vi "Read Debug Data.vi"(8 "error in (no error)":errorcluster, 11 "Debugger In":refnum<class "Debugger.lvclass">) -> (0 "error out":errorcluster, 2 "Data Log":refnum<class "Debug Data.lvclass">[](array[class]), 3 "Debugger Out":refnum<class "Debugger.lvclass">)   [LabVIEW 2020, in "Debugger.lvclass"]
uses:
  Debugger.lvclass
  Debug Data/Debug Data.lvclass
  Debug Log/Debug Log.lvclass/Debug Log.ctl
  Debug Log/Read Unfiltered Log Content.vi
  Filter/Filter.lvclass
  Debugger.lvclass/Debugger.ctl
  Debug Log/Debug Log.lvclass
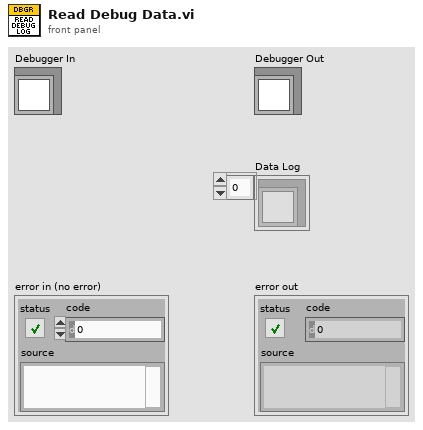
[diagram p1: front panel]
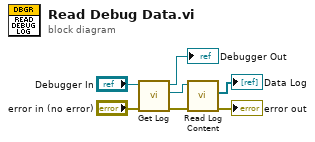
[diagram p0: block diagram]
diagram:
  n1 = call "Get Log.vi"("error in (no error)"="error in (no error)", "Debugger in"="Debugger In") -> ("error out"=w3:errorcluster, "Log"=w7:refnum<class "Debug Log.lvclass">, "Debugger out"=→"Debugger Out":refnum<class "Debugger.lvclass">)  [unwired: 7 in]
  n2 = call "Read Log Content.vi"("error in (no error)"=w3, "Debug Log In"=w7) -> ("error out"=→"error out":errorcluster, "Data Log"=→"Data Log":refnum<class "Debug Data.lvclass">[])  [unwired: 7 in, 1 out]
